vi "strings to memory.vi"(8 "error in":errorcluster, 11 "1.0.0":T1) -> (0 "error out":errorcluster, 3 "memory hierarchy":T5)   [LabVIEW 2023, in "CEF.lvlib"]
doc: "Unflattens a flattened instance data hierarchy into an object hierarchy.Copyright 2017 National Instruments Corporation\n\nLicensed under the Apache License, Version 2.0 (the \"License\"); you may not use this file except in compliance with the License. You may obtain a copy of the License at http://www.apache.org/licenses/LICENSE-2.0\nUnless required by applicable law or agreed to in writing, software distributed under the License is distributed on an \"AS IS\" BASIS, WITHOUT WARRANTIES OR CONDITIONS OF ANY KIND, either express or implied. See the License for the specific language governing permissions and limitations under the License."
uses:
  CEF.lvlib
  hierarchy repo/memory hierarchy.ctl
  hierarchy repo/full hierarchy.ctl
  hierarchy element.ctl
  serializable configuration/CEF_serializable configuration.lvclass
  flat hierarchy.ctl
  instance data.ctl
  class discovery singleton/class discovery singleton methods.ctl
  hierarchy repo/CEF_HierarchyRepo.lvclass
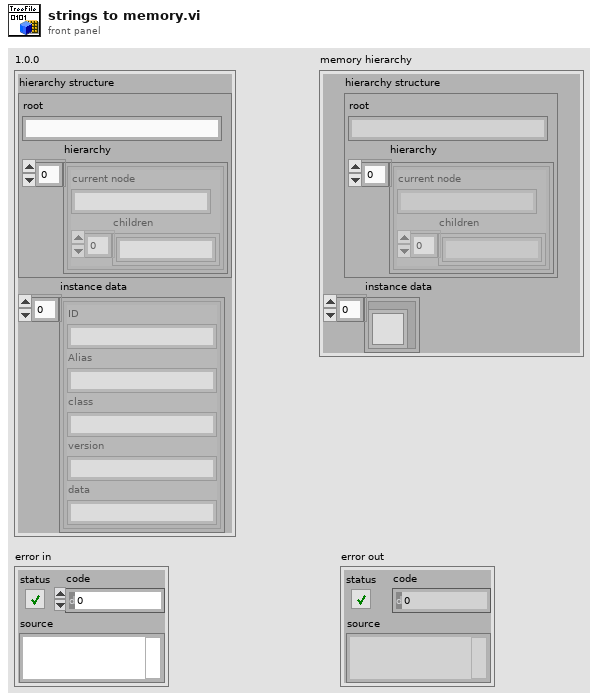
[diagram p1: front panel]
types:
  T1 = typedef "CEF.lvlib/flat hierarchy.ctl" = cluster{"hierarchy structure":T2, "instance data":T4[]}
  T2 = typedef "CEF.lvlib/CEF_HierarchyRepo.lvclass/full hierarchy.ctl" = cluster{"root":string, "hierarchy":T3[]}
  T3 = typedef "CEF.lvlib/hierarchy element.ctl" = cluster{"current node":string, "children":string[]}
  T4 = typedef "CEF.lvlib/instance data.ctl" = cluster{"ID":string, "Alias":string, "class":string, "version":string, "data":string}
  T5 = typedef "CEF.lvlib/CEF_HierarchyRepo.lvclass/memory hierarchy.ctl" = cluster{"hierarchy structure":T2, "instance data":refnum<class "CEF_serializable configuration.lvclass">[]}
  T6 = typedef "CEF.lvlib/class discovery singleton methods.ctl" = enum16{"add search paths", "load class by name", "list available classes", "get class path", "delete cache"}
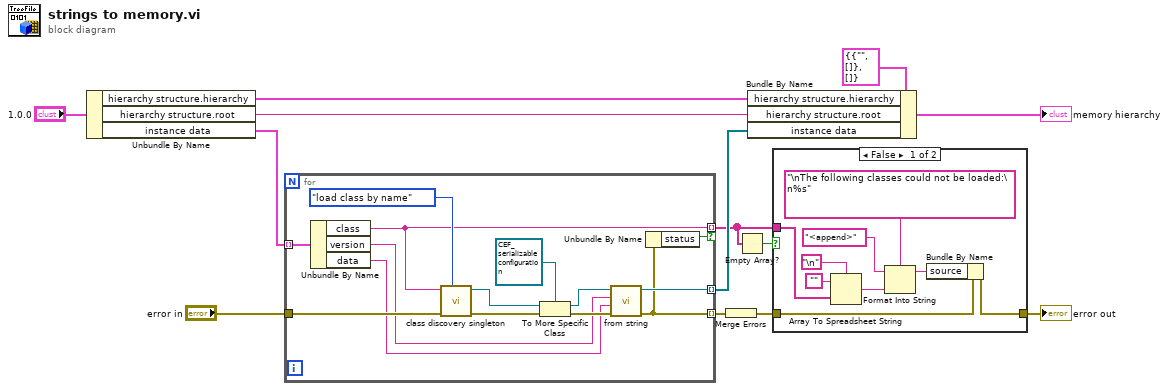
[diagram p0: block diagram]
diagram:
  n1 = Unbundle By Name("1.0.0") -> ("hierarchy structure.hierarchy"=w9:T3[], "hierarchy structure.root"=w10:string, "instance data"=w8:T4[])
  n2 = for {
    tunnel: w8 -> [w27] mode=indexing
    tunnel: [w21] -> w6 mode=indexing
    tunnel: "error in" -> [w24]
    tunnel: [w18] -> w5 mode=indexing
    tunnel: [w15] -> w1 mode=indexing if=w17
    n3 = Unbundle By Name(w27) -> ("class"=w15:string, "version"=w19:string, "data"=w20:string)
    n4 = call "class discovery singleton.vi"("method"=class_discovery_singleton_methods."load class by name", "error in"=w24, "Class Name"=w15) -> ("error out"=w26:errorcluster, "LabVIEW Object"=w14:refnum<class>)  [unwired: 5 in, 2 out]
    n5 = To More Specific Class(target class=refnum<class "CEF_serializable configuration.lvclass"> refnum ("configuration in"), reference=w14, error in=w26) -> (specific class reference=w22:refnum<class "CEF_serializable configuration.lvclass">, error out=w23:errorcluster)
    n6 = call-dynamic "from string.vi"("error in"=w23, "data"=w20, "version"=w19, "CEF_Configuration in"=w22) -> ("error out"=w18:errorcluster, "CEF_Configuration out"=w21:refnum<class "CEF_serializable configuration.lvclass">)  [unwired: 6 in]
    n7 = Unbundle By Name(w18) -> ("status"=w17:bool)
  }
  n8 = Merge Errors(w5) -> (w3:errorcluster)
  n9 = Empty Array?(array=w1) -> (empty?=w4:bool)
  n10 = Bundle By Name(cluster=T5 {"hierarchy structure"={"root"="", "hierarchy"=[]}, "instance data"=[]} ("memory hierarchy"), "hierarchy structure.hierarchy"=w9, "hierarchy structure.root"=w10, "instance data"=w6) -> (→"memory hierarchy":T5)
  n11 = case shown="False" w4 {
    tunnel: w3 -> [w36 w37]
    tunnel: [w35 w37] -> w2
    tunnel: w1 -> [w29 _]
    frame False {
      n12 = Array To Spreadsheet String(delimiter (Tab)="\n", array=w29, 3:"" ("format string")) -> (spreadsheet string=w31:string)
      n13 = Format Into String(format string="\nThe following classes could not be loaded:\n%s", initial string="<append>", w31) -> (resulting string=w30:string)  [unwired: 1 in, 1 out]
      n14 = Bundle By Name(cluster=w36, "source"=w30) -> (w35:errorcluster)
    }
    frame True {
    }
  }
  "error out" <- w2
